vi "Chi-Squared Moments.vi"(10 "k":i32=1) -> (0 "error":i32, 2 "variance":dbl=2.0, 3 "mean":dbl=1.0)   [LabVIEW 2014, in "NI_Gmath.lvlib"]
doc: "Returns the expected mean and variance of the random variate X, where X describes the selected distribution type. You must manually select the polymorphic instance to use."
uses:
  NI_Gmath.lvlib
  st_error_code.ctl
panel:
  # "Chi-Squared Moments"
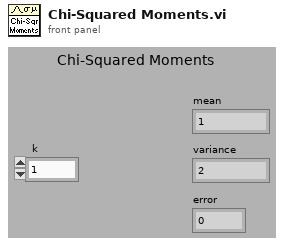
[diagram p1: front panel]
types:
  T1 = typedef "NI_Gmath.lvlib/st_error_code.ctl" = i32
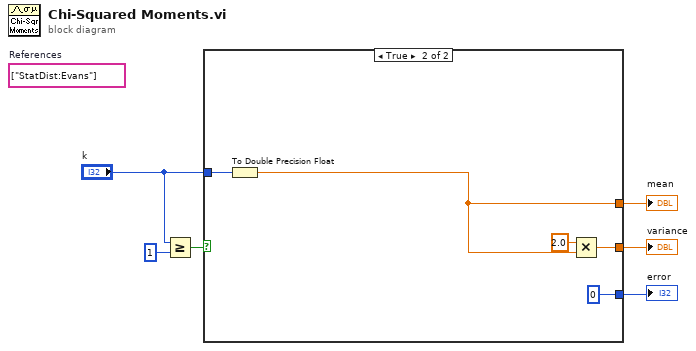
[diagram p0: block diagram]
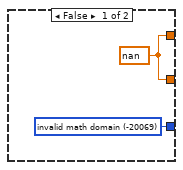
[diagram p2: hidden frame]
diagram:
  (unwired) string[] ["StatDist:Evans"]  # References
  n1 = Greater Or Equal?(x="k", y=1) -> (x >= y?=w2:bool)
  n2 = case shown="True" w2 {
    tunnel: [w7 0 ("invalid math domain")] -> w6
    tunnel: [w8 w9] -> w5
    tunnel: "k" -> [_ w12]
    tunnel: [w8 w10] -> w1
    frame False {
      w7 = T1 -20069 items=["invalid math domain"=-20069, "Fourier interpolation size m >= n"=-20070, "empty array"=-20003] ("stat interp error code")
      w8 = nan
    }
    frame True {
      n3 = To Double Precision Float(number=w12) -> (double precision float=w9:dbl)
      n4 = Multiply(x=2.0, y=w9) -> (x*y=w10:dbl)
    }
  }
  "mean" <- w5
  "error" <- w6
  "variance" <- w1
